vi "Protocol.Address Lookup Table.vi"(7 "Action":T3, 8 "error in (no error)":errorcluster, 9 "Address":u8, 10 "Data":T2 {"Name" format="%.0x"}, 11 "Address LUT":T1) -> (0 "error out":errorcluster, 1 "All Data":T2[](array[typedef]) {"Name" format="%.0x"}, 2 "Data":T2 {"Name" format="%.0x"}, 3 "Address LUT out":T1, 4 "Found?":bool)   [LabVIEW 2015, in "J1939 Addon Engine.lvlib"]
uses:
  J1939 Addon Engine.lvlib
  Shared/Types/Address Lookup Table Data.ctl
  Types/Protocol.Address Lookup Table Action.ctl
  Types/Protocol.Address Table Reference.ctl
  Shared/J1939 Addon Shared.lvlib
panel:
  # "OUTPUTS"
  # "INPUTS"
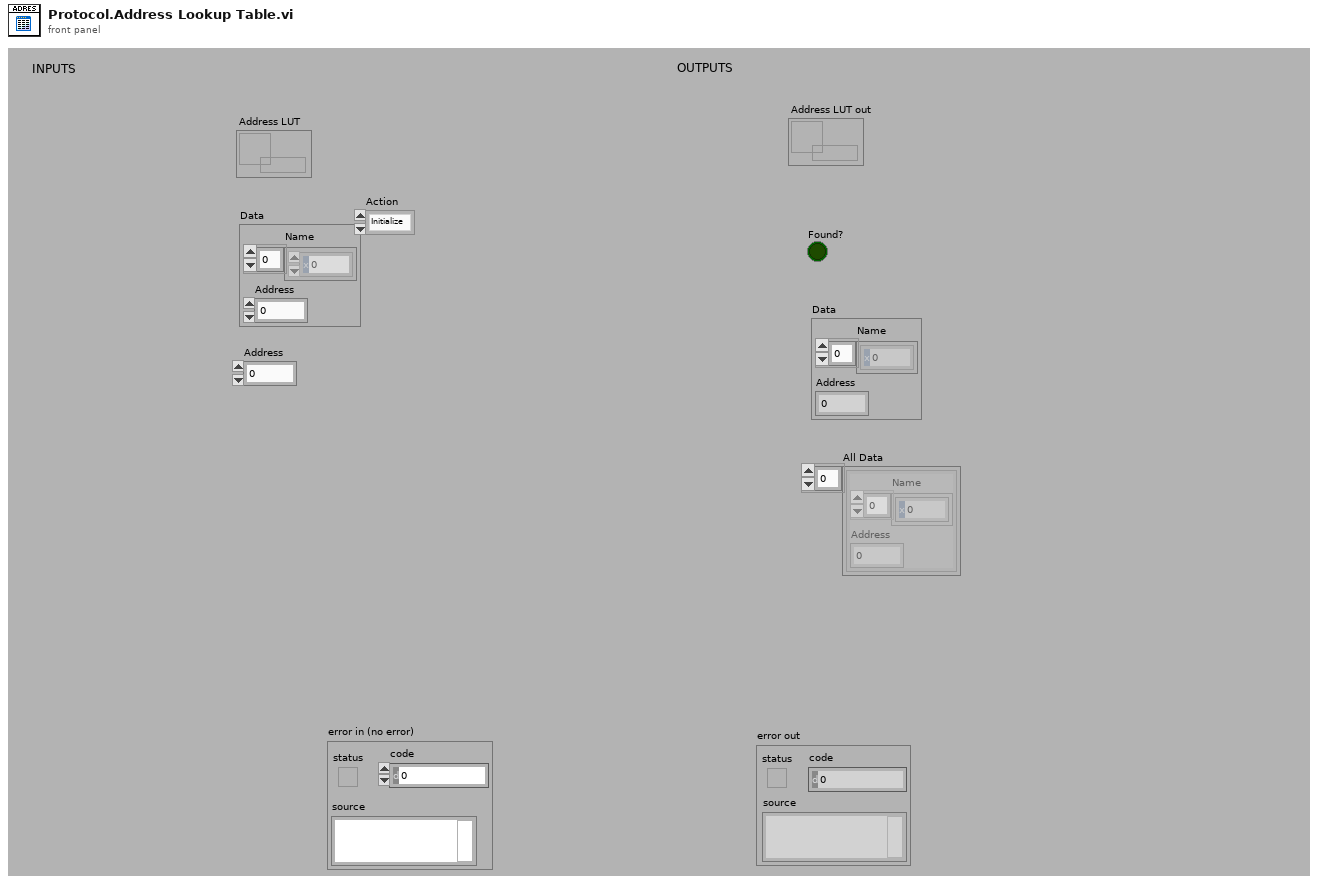
[diagram p1: front panel]
types:
  T1 = typedef "J1939 Addon Engine.lvlib/Protocol.Address Table Reference.ctl" = refnum<data-value>
  T2 = typedef "J1939 Addon Shared.lvlib/Address Lookup Table Data.ctl" = cluster{"Name":u8[], "Address":u8}
  T3 = typedef "J1939 Addon Engine.lvlib/Protocol.Address Lookup Table Action.ctl" = enum16{"Initialize", "Add", "Get", "Remove", "Get All"}
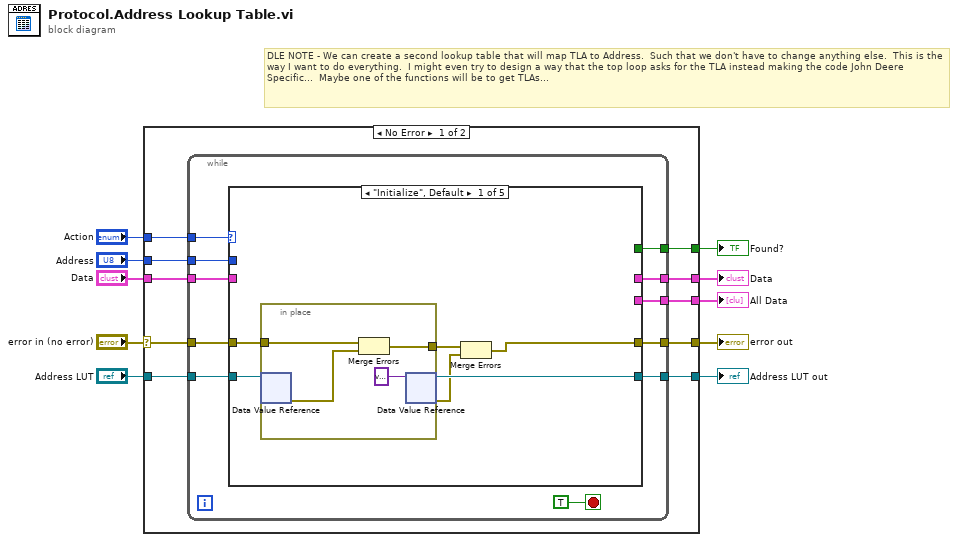
[diagram p0: block diagram]
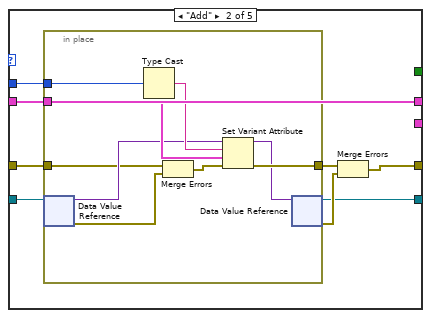
[diagram p2: hidden frame]
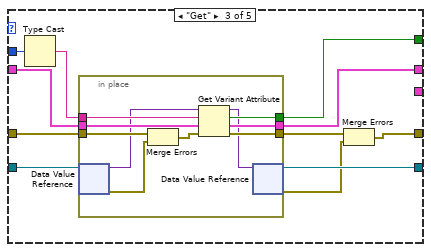
[diagram p3: hidden frame]
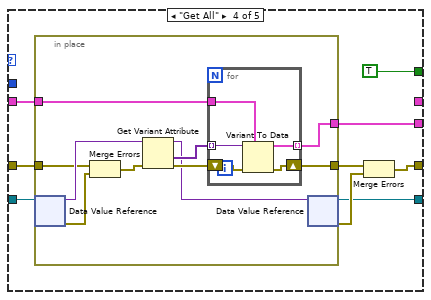
[diagram p4: hidden frame]
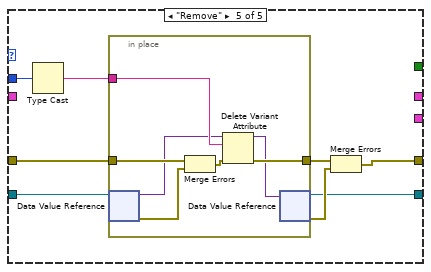
[diagram p5: hidden frame]
diagram:
  # "DLE NOTE - We can create a second lookup table that will map TLA to Address.  Such that we don't have to change anything else.  This is the way I want to do everything.  I might even try to design a way that the top loop asks for the TLA instead making the code John Deere Specific...  Maybe one of the functions will be to get TLAs..."
  n1 = case shown="No Error" "error in (no error)" {
    selector: "error in (no error)" -> [w16 w120]
    tunnel: [w15 w120] -> w9
    tunnel: "Data" -> [w19 _]
    tunnel: "Action" -> [w20 _]
    tunnel: [w18 _] -> w6
    tunnel: "Address" -> [w17 _]
    tunnel: [w14 _] -> w4
    tunnel: [w13 _] -> w3
    tunnel: "Address LUT" -> [w12 w119]
    tunnel: [w11 w119] -> w1
    frame No Error {
      n2 = while {
        tunnel: w20 -> [w31]
        tunnel: w19 -> [w24]
        tunnel: [w29] -> w18
        tunnel: w17 -> [w28]
        tunnel: w16 -> [w27]
        tunnel: [w26] -> w15
        tunnel: [w25] -> w14
        tunnel: [w23] -> w13
        tunnel: w12 -> [w22]
        tunnel: [w21] -> w11
        stop <- TRUE stop-if-true
        n3 = case shown="\"Initialize\", Default" w31 {
          tunnel: [_ w49 w65 _ _] -> w29
          tunnel: w28 -> [_ w48 w69 _ w111]
          tunnel: w27 -> [w35 w47 w67 w88 w110]
          tunnel: [w32 w44 w60 w82 w106] -> w26
          tunnel: [_ _ w64 TRUE _] -> w25
          tunnel: w24 -> [_ w49 w66 w86 _]
          tunnel: [_ _ _ w85 _] -> w23
          tunnel: w22 -> [w37 w46 w63 w84 w108]
          tunnel: [w36 w42 w62 w80 w104] -> w21
          frame "Initialize", Default {
            n4 = in-place {
              in-place-border: w35 -> [w40]
              in-place-border: [w38] -> w34
              n5 = in-place-dvr #1(w37) -> (w39:errorcluster)  [unwired: 1 out]
              n6 = Merge Errors(w40, w39) -> (w38:errorcluster)
              n7 = in-place-dvr #1(variant ("duplicate variant")) -> (w36:T1, w33:errorcluster)
            }
            n8 = Merge Errors(w34, w33) -> (w32:errorcluster)
          }
          frame "Add" {
            n9 = in-place {
              in-place-border: w49 -> [w58]
              in-place-border: w48 -> [w57]
              in-place-border: w47 -> [w51]
              in-place-border: [w55] -> w43
              n10 = in-place-dvr #2(w46) -> (w54:variant, w52:errorcluster)
              n11 = Type Cast(x=w57) -> (*(type *) &x=w56:string)  [unwired: 1 in]
              n12 = Merge Errors(w51, w52) -> (w50:errorcluster)
              n13 = Set Variant Attribute(Variant=w54, name=w56, value=w58, error in=w50) -> (Variant out=w53:variant, error out=w55:errorcluster)  [unwired: 1 out]
              n14 = in-place-dvr #2(w53) -> (w42:T1, w45:errorcluster)
            }
            n15 = Merge Errors(w43, w45) -> (w44:errorcluster)
          }
          frame "Get" {
            n16 = Type Cast(x=w69) -> (*(type *) &x=w68:string)  [unwired: 1 in]
            n17 = in-place {
              in-place-border: w68 -> [w79]
              in-place-border: w67 -> [w78]
              in-place-border: [w77] -> w59
              in-place-border: w66 -> [w76]
              in-place-border: [w75] -> w65
              in-place-border: [w74] -> w64
              n18 = in-place-dvr #3(w63) -> (w73:variant, w70:errorcluster)
              n19 = Merge Errors(w78, w70) -> (w71:errorcluster)
              n20 = Get Variant Attribute(Variant=w73, name=w79, default value (empty Variant)=w76, error in=w71) -> (duplicate Variant=w72:variant, found=w74:bool, value=w75:T2, error out=w77:errorcluster)
              n21 = in-place-dvr #3(w72) -> (w62:T1, w61:errorcluster)
            }
            n22 = Merge Errors(w59, w61) -> (w60:errorcluster)
          }
          frame "Get All" {
            n23 = in-place {
              in-place-border: w88 -> [w90]
              in-place-border: w86 -> [w97]
              in-place-border: [w95] -> w81
              in-place-border: [w94] -> w85
              n24 = in-place-dvr #4(w84) -> (w93:variant, w91:errorcluster)
              n25 = Merge Errors(w90, w91) -> (w89:errorcluster)
              n26 = Get Variant Attribute(Variant=w93, error in=w89) -> (duplicate Variant=w92:variant, values=w98:variant[], error out=w96:errorcluster)  [unwired: 2 in, 1 out]
              n27 = for {
                tunnel: w98 -> [w103] mode=indexing
                tunnel: w97 -> [w102]
                shift-right: [w100] -> w95
                shift-left: w96 -> [w101]
                tunnel: [w99] -> w94 mode=indexing
                n28 = Variant To Data(error in=w101, type=w102, Variant=w103) -> (data=w99:T2, error out=w100:errorcluster)
              }
              n29 = in-place-dvr #4(w92) -> (w80:T1, w83:errorcluster)
            }
            n30 = Merge Errors(w81, w83) -> (w82:errorcluster)
          }
          frame "Remove" {
            n31 = Type Cast(x=w111) -> (*(type *) &x=w109:string)  [unwired: 1 in]
            n32 = in-place {
              in-place-border: w110 -> [w118]
              in-place-border: [w117] -> w105
              in-place-border: w109 -> [w116]
              n33 = in-place-dvr #5(w108) -> (w115:variant, w112:errorcluster)
              n34 = Merge Errors(w118, w112) -> (w113:errorcluster)
              n35 = Delete Variant Attribute(4:w113, 6:w116, 7:w115) -> (0:w117:errorcluster, 3:w114:variant)  [unwired: 1 out]
              n36 = in-place-dvr #5(w114) -> (w104:T1, w107:errorcluster)
            }
            n37 = Merge Errors(w105, w107) -> (w106:errorcluster)
          }
        }
      }
    }
    frame Error {
    }
  }
  "error out" <- w9
  "Data" <- w6
  "Found?" <- w4
  "All Data" <- w3
  "Address LUT out" <- w1
